vi "Run_Task.vi"(8 "error in (no error)":errorcluster caption="entrée d'erreur (pas d'erreur)", 11 "Class Log_File Altyor en entrée":refnum<class "Class Log_File Altyor.lvclass">) -> (0 "error out":errorcluster caption="sortie d'erreur", 3 "Class Log_File Altyor en sortie":refnum<class "Class Log_File Altyor.lvclass">)   [LabVIEW 2020, in "Library Instrument & Equipement.lvlib" / "Library Log_File.lvlib" / "Class Log_File Altyor.lvclass"]
uses:
  Class Log_File Altyor.lvclass
  C:/Users/ngarcin/OneDrive - Altyor/Standard TB/Class/Log File/Log_File (Default)/Class Log_File (Default).lvclass
  Task_LogFile.vi
  Read CSV File/CSV_File (Default)/Class CSV_File.lvclass
  Class Log_File Altyor.lvclass/Class Log_File Altyor.ctl
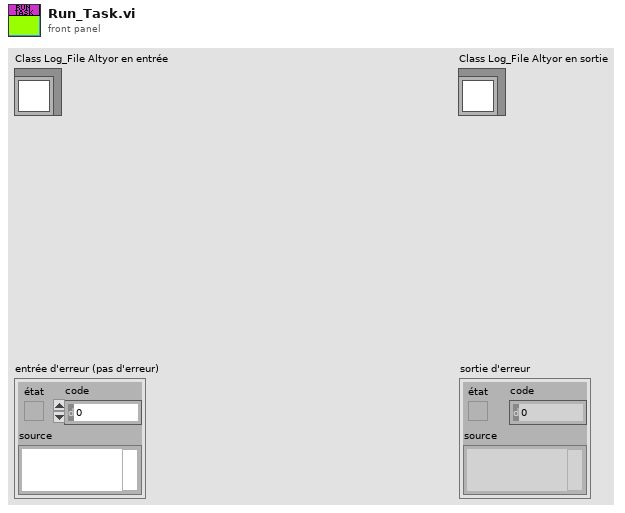
[diagram p1: front panel]
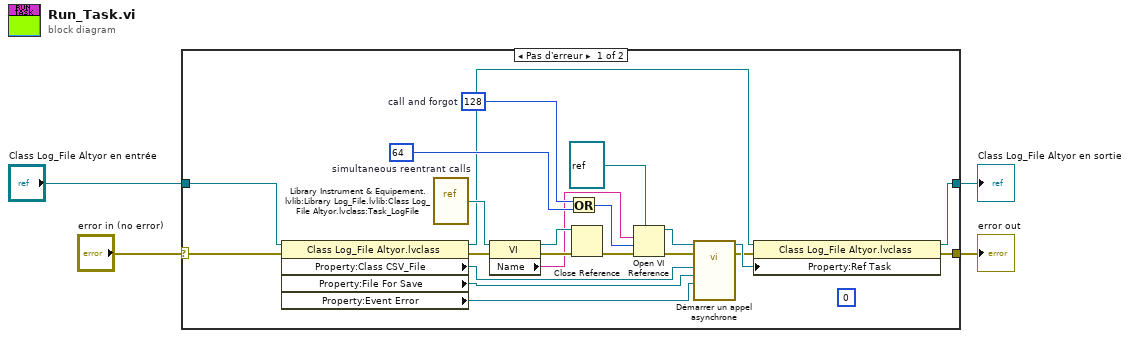
[diagram p0: block diagram]
diagram:
  n1 = case shown="Pas d'erreur" "error in (no error)" {
    selector: "error in (no error)" -> [w12 w28]
    tunnel: [w5 w28] -> w2
    tunnel: "Class Log_File Altyor en entrée" -> [w10 w27]
    tunnel: [w8 w27] -> w1
    frame No Error {
      (unwired) 0 ("options")
      w22 = 64  # simultaneous reentrant calls
      w21 = 128  # call and forgot
      n2 = property class="Class Log_File Altyor.lvclass"(reference=w10, error in=w12) -> (reference out=w9:refnum<class "Class Log_File Altyor.lvclass">, error out=w11:errorcluster, "Property:Class CSV_File"=w15:refnum<class "Class CSV_File.lvclass">, "Property:File For Save"=w14:refnum<queue>, "Property:Event Error"=w13:refnum<user-event>)
      n3 = vi-ref "Library Instrument & Equipement.lvlib:Library Log_File.lvlib:Class Log_File Altyor.lvclass:Task_LogFile.vi"() -> (w24:refnum<vi>)
      n4 = property class="VI"(reference=w24, error in=w11) -> (reference out=w26:refnum<vi>, error out=w25:errorcluster, "Name"=w18:string)
      n5 = Or(x=w21, y=w22) -> (x .or. y?=w19:i32)
      n6 = Close Reference(reference=w26, error in (no error)=w25) -> (error out=w20:errorcluster)
      n7 = Open VI Reference(type specifier VI Refnum (for type only)=refnum<vi> refnum ("spécificateur de type du refnum de VI (pour type seulement)"), vi path=w18, options=w19, error in (no error)=w20) -> (vi reference=w17:refnum<vi>, error out=w16:errorcluster)  [unwired: 2 in]
      n8 = call-by-ref "Démarrer un appel asynchrone"(reference=w17, error in=w16, "Event Error"=w13, "File For Save"=w14, "Class CSV_File"=w15) -> (reference out=w7:refnum<vi>, error out=w6:errorcluster)  [unwired: 9 in]
      n9 = property class="Class Log_File Altyor.lvclass"(reference=w9, error in=w6, "Property:Ref Task"=w7) -> (reference out=w8:refnum<class "Class Log_File Altyor.lvclass">, error out=w5:errorcluster)
    }
    frame Error {
    }
  }
  "error out" <- w2
  "Class Log_File Altyor en sortie" <- w1
